vi "dsyr2k - Symmetric Matrix Rank-2k Update (DBL).vi"(4 "beta":dbl=1.0, 6 "alpha":dbl=1.0, 7 "operation":T2 items=["Direct", "Conjugated & Transposed", "Transposed"], 8 "matrix C type":T1=3 items=["Lower Triangular"=2, "Upper Triangular"=3], 9 "C":T3, 10 "B":T3, 11 "A":T3) -> (0 "error":i32, 3 "dsyr2k":T3)   [LabVIEW 2017, in "NI_AALBLAS.lvlib"]
doc: "Calculates the rank-2k update of a symmetric matrix."
uses:
  NI_AALBLAS.lvlib
  RealMatrix.ctl
  LV_Transpose.ctl
  LV_UpLo.ctl
  Fucntion.ctl
  Order.ctl
  BLAS3 Utility(DBL).vi
  NI_Matrix.lvlib
panel:
  # "dsyr2k=alpha*A*B'+alpha*B*A'+beta*C / dsyr2k=alpha*A'*B+alpha*B'*A+beta*C"
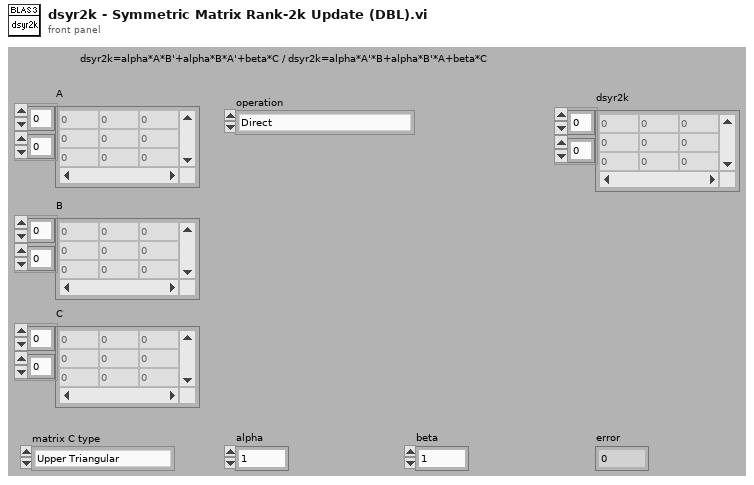
[diagram p1: front panel]
types:
  T1 = typedef "NI_AALBLAS.lvlib/LV_UpLo.ctl" = i32
  T2 = typedef "NI_AALBLAS.lvlib/LV_Transpose.ctl" = i32
  T3 = typedef "NI_Matrix.lvlib/RealMatrix.ctl" = dbl[][]
  T4 = typedef "NI_AALBLAS.lvlib/Order.ctl" = i32
  T5 = typedef "NI_AALBLAS.lvlib/Fucntion.ctl" = u16
  T6 = typedef "NI_AALBLAS.lvlib/Operation_Transpose.ctl" = i32
  T7 = typedef "NI_AALBLAS.lvlib/UpLo.ctl" = i32
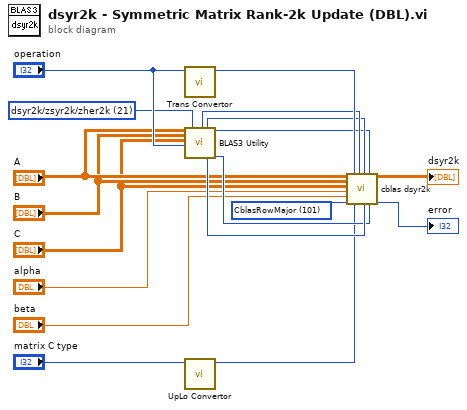
[diagram p0: block diagram]
diagram:
  w1 = T4 101 items=["CblasRowMajor"=101, "CblasColMajor"=102] ("order")
  w5 = T5 21 items=["ddot/zdotu/zdotc", "daxpy/zaxpy", "dnrm2/dznrm2", "dasum/dzasum", "dcopy/zcopy", "dswap/zswap", "drotm", "drot/zdrot", "idamax/izamax", "idamin/izamin", "dgemv/zgemv", "dsymv/zhemv", "dtrmv/ztrmv", "dsyr/zher", "dsyr2/zher2", "dger/zgeru/zgerc", "dtrsv/ztrsv", "dgemm/zgemm", "dsymm/zsymm/zhemm", "dtrmm/ztrmm", "dsyrk/zsyrk/zherk", "dsyr2k/zsyr2k/zher2k", "dtrsm/ztrsm"] ("function")
  n1 = call "Trans Convertor.vi"("operation"="operation") -> ("trans"=w11:T6)  [unwired: 10 out]
  n2 = call-poly "BLAS3 Utility.vi"("A"="A", "B/X"="B", "C"="C", "operation A"="operation", "function"=w5) -> ("lda"=w4:i32, "ldb/ldx"=w3:i32, "n"=w17:i32, "ldc"=w2:i32, "k"=w16:i32)  [unwired: 1 in, 9 out]
  n3 = call "UpLo Convertor.vi"("triangle matrix type"="matrix C type") -> ("uplo"=w12:T7)  [unwired: 10 out]
  n4 = call "cblas dsyr2k.vi"("A"="A", "B"="B", "C"="C", "alpha"="alpha", "beta"="beta", "order"=w1, "trans"=w11, "uplo"=w12, "lda"=w4, "ldb"=w3, "n"=w17, "ldc"=w2, "k"=w16) -> ("dsyr2k"=→"dsyr2k":T3, "error"=→"error":i32)  [unwired: 5 out]
